vi "Convert VI Libraries to Dirs (proxy)__ogtk.vi"(4 "backup vi libraries":bool, 6 "automatically rename":bool, 8 "error in (no error)":errorcluster, 9 "multiplatform names":bool, 10 "dir name scheme (0:remove .llb)":enum16{"remove .llb", "same name", "prompt"}(ring), 11 "VI libraries":path[](array[path])) -> (0 "error out":errorcluster, 1 "destination paths":path[](array[path]), 2 "renamed VIs original name":string[](array[string]), 3 "renamed VIs new path":path[](array[path]))   [LabVIEW 2012]
doc: "Converts an array of VI Libraries (.llb) into Directories. \n\nNote: This VI dynamically calls the LabVIEW subVI \"Convert VI Libraries to Dirs.vi\" located at <LabVIEW>\\project\\llbedit.llb (as it is not in the VI search paths)."
panel:
  in  "type specifier":refnum<vi>
  # "Convert VI Libraries to Dirs (proxy).vi\n\nCalls \"Convert VI Libraries to Dirs.vi\" by reference\n\nPlease visit http://www.OpenG.org to learn about the\nOpen Source LabVIEW software movement.\n\nNOTICE -- YOU MUST LEAVE THIS NOTICE IN PLACE.  PER THE TERMS OF THE LICENSE BELOW, YOU MAY SUBLICENSE THIS SOFTWARE \nIN ANY WAY THAT DOES NOT CONFLICT WITH THIS LICENSE.\n\n### BSD License (http://www.opensource.org/licenses/bsd-license.php) Begin ###\n \nCopyright (c) 2003, Jim Kring <jim@jimkring.com>\n\nAll rights reserved.\n\nRedistribution and use in source and binary forms, with or without modification, are permitted provided that the following conditions are met:\n\n    * Redistributions of source code must retain the above copyright notice, this list of conditions and the following disclaimer.\n    * Redistributions in binary form must reproduce the above copyright notice, this list of conditions and the following disclaimer in the \n       documentation and/or other materials provided with the distribution.\n    * Neither the name of SciWare, James Kring, Inc., nor the names of its contributors may be used to endorse or promote products derived \n       from this software without specific prior written permission.\n\nTHIS SOFTWARE IS PROVIDED BY THE COPYRIGHT HOLDERS AND CONTRIBUTORS \"AS IS\" AND ANY EXPRESS OR IMPLIED WARRANTIES, \nINCLUDING, BUT NOT LIMITED TO, THE IMPLIED WARRANTIES OF MERCHANTABILITY AND FITNESS FOR A PARTICULAR PURPOSE ARE \nDISCLAIMED. IN NO EVENT SHALL THE COPYRIGHT OWNER OR CONTRIBUTORS BE LIABLE FOR ANY DIRECT, INDIRECT, INCIDENTAL,\n SPECIAL, EXEMPLARY, OR CONSEQUENTIAL DAMAGES (INCLUDING, BUT NOT LIMITED TO, PROCUREMENT OF SUBSTITUTE GOODS OR \nSERVICES; LOSS OF USE, DATA, OR PROFITS; OR BUSINESS INTERRUPTION) HOWEVER CAUSED AND ON ANY THEORY OF LIABILITY, \nWHETHER IN CONTRACT, STRICT LIABILITY, OR TORT (INCLUDING NEGLIGENCE OR OTHERWISE) ARISING IN ANY WAY OUT OF THE USE \nOF THIS SOFTWARE, EVEN IF ADVISED OF THE POSSIBILITY OF SUCH DAMAGE.\n\n### BSD License End ###"
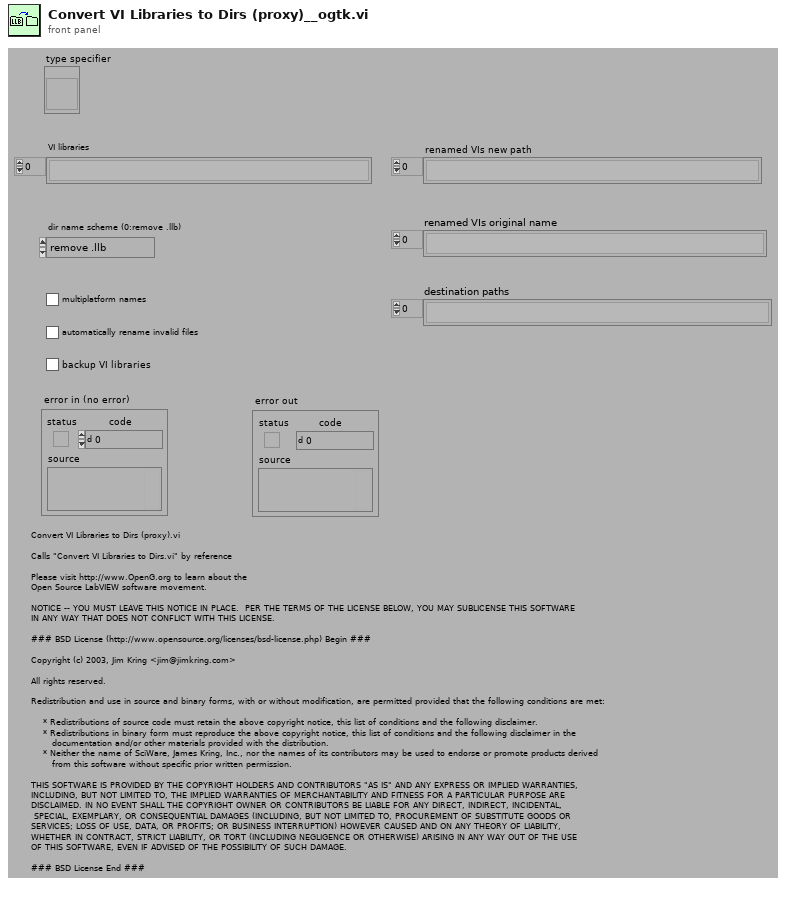
[diagram p1: front panel]
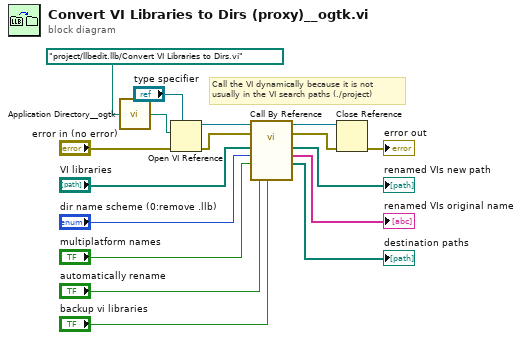
[diagram p0: block diagram]
diagram:
  # "Call the VI dynamically because it is not\nusually in the VI search paths (./project)"
  n1 = call <userlib>:"Application Directory__ogtk.vi"("Relative path (.)"=path "project/llbedit.llb/Convert VI Libraries to Dirs.vi") -> ("Application Directory (+ Relative)"=w10:path)
  n2 = Open VI Reference(type specifier VI Refnum (for type only)="type specifier", vi path=w10, error in (no error)="error in (no error)") -> (vi reference=w16:refnum<vi>, error out=w9:errorcluster)  [unwired: 3 in]
  n3 = call-by-ref "?"(reference=w16, error in=w9, "backup vi libraries"="backup vi libraries", "automatically rename"="automatically rename", "multiplatform names"="multiplatform names", "dir name scheme (0:remove .llb)"="dir name scheme (0:remove .llb)", "VI libraries"="VI libraries") -> (reference out=w15:refnum<vi>, error out=w14:errorcluster, "destination paths"=→"destination paths":path[], "renamed VIs original name"=→"renamed VIs original name":string[], "renamed VIs new path"=→"renamed VIs new path":path[])  [unwired: 4 in]
  n4 = Close Reference(reference=w15, error in (no error)=w14) -> (error out=→"error out":errorcluster)
